vi "Total DAQ Link Data.vi"(9 "2 LBCB Archiving Mode":bool, 10 "Use Hold":bool, 11 "Number of LBCBs":T1) -> (1 "External Sensors":dbl[](array[numeric]), 2 "Act Data":dbl[](array[numeric]), 3 "Cart Data":dbl[](array[numeric]))   [LabVIEW 2009]
uses:
  Data Access Objects/Application/Number Of LBCBs.ctl
  Cartesian Measurment Actions.ctl
  Data Access Objects/Metadata/LBCB Number.ctl
  Data Access Objects/Metadata/DAO Actions.ctl
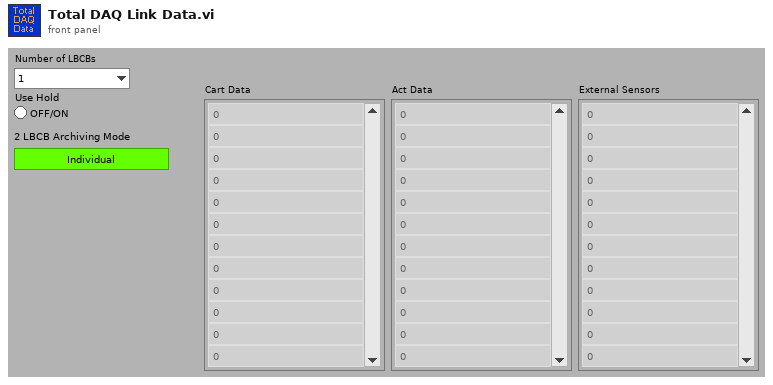
[diagram p1: front panel]
types:
  T1 = typedef "Number Of LBCBs.ctl" = enum16{"1", "2"}
  T2 = typedef "Cartesian Measurment Actions.ctl" = enum16{"Set Data", "Get", "Init", "Set Offsets"}
  T3 = typedef "LBCB Number.ctl" = enum16{"LBCB1", "LBCB2"}
  T4 = typedef "DAO Actions.ctl" = enum16{"Init", "Get", "Set"}
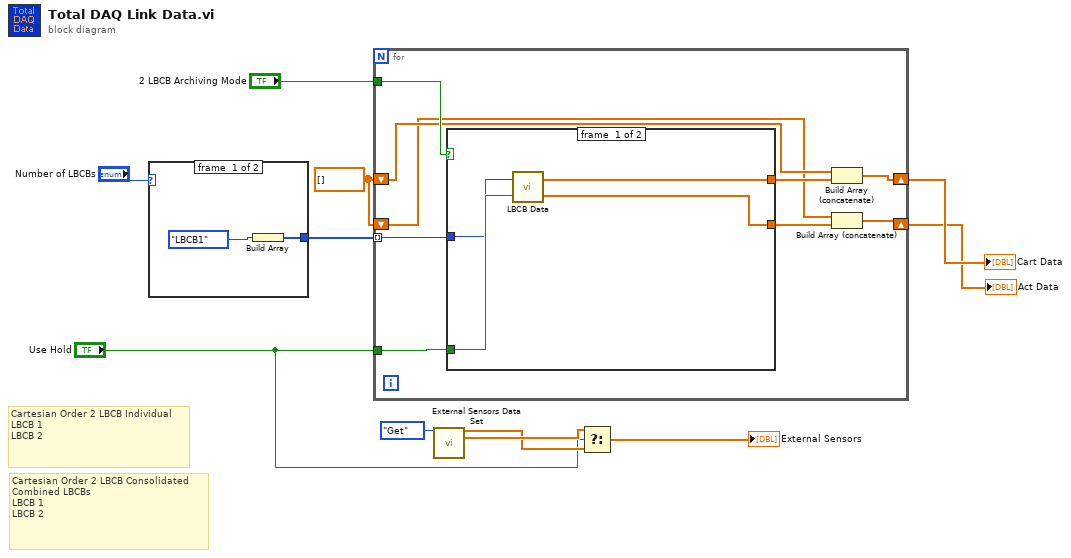
[diagram p0: block diagram]
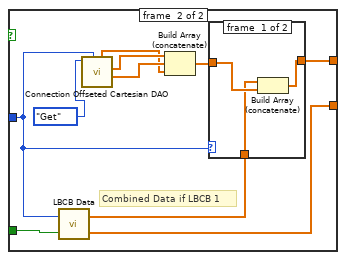
[diagram p2: hidden frame]
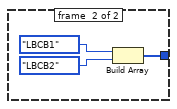
[diagram p4: hidden frame]
diagram:
  w8 = dbl[] [] ("Cart Data")
  # "Cartesian Order 2 LBCB Consolidated\nCombined LBCBs\nLBCB 1\nLBCB 2"
  # "Cartesian Order 2 LBCB Individual\nLBCB 1\nLBCB 2"
  n1 = case shown="\"1\", Default" "Number of LBCBs" {
    tunnel: [w12 w14] -> w10
    frame #0 {
      n2 = Build Array(LBCB_Number."LBCB1" ("LBCB Number")) -> (w12:T3[])
    }
    frame #1 {
      n3 = Build Array(LBCB_Number."LBCB1" ("LBCB Number"), LBCB_Number."LBCB2" ("LBCB Number")) -> (w14:T3[])
    }
  }
  n4 = for {
    tunnel: w10 -> [w23] mode=indexing
    tunnel: "Use Hold" -> [w25]
    tunnel: "2 LBCB Archiving Mode" -> [w21]
    shift-right: [w20] -> w7
    shift-left: w8 -> [w19]
    shift-right: [w18] -> w6
    shift-left: w8 -> [w17]
    n5 = case shown="True" w21 {
      tunnel: w25 -> [w29 w39]
      tunnel: [w28 w38] -> w24
      tunnel: w23 -> [w27 w33]
      tunnel: [w26 w30] -> w22
      frame #0 {
        n6 = call "LBCB Data.vi"("Use Hold"=w29, "LBCB Number"=w27) -> ("Act Data"=w28:dbl[], "Cart Data"=w26:dbl[])
      }
      frame #1 {
        # "Combined Data if LBCB 1"
        n7 = call "LBCB Data.vi"("Use Hold"=w39, "LBCB Number"=w33) -> ("Act Data"=w38:dbl[], "Cart Data"=w31:dbl[])
        n8 = call "Connection Offseted Cartesian DAO.vi"("LBCB Number"=w33, "DAO Actions"=DAO_Actions."Get") -> ("CO Disp Out"=w35:dbl[], "CO Cmd Out"=w36:dbl[], "CO Forces Out"=w34:dbl[])  [unwired: 6 in, 1 out]
        n9 = Build Array (concatenate)(w36, w35, w34) -> (w32:dbl[])
        n10 = case shown="\"LBCB1\"" w33 {
          tunnel: w32 -> [w42 w43]
          tunnel: w31 -> [w41 _]
          tunnel: [w40 w43] -> w30
          frame #0 {
            n11 = Build Array (concatenate)(w41, w42) -> (w40:dbl[])
          }
          frame #1 {
          }
        }
      }
    }
    n12 = Build Array (concatenate)(w19, w22) -> (w20:dbl[])
    n13 = Build Array (concatenate)(w17, w24) -> (w18:dbl[])
  }
  "Cart Data" <- w7
  "Act Data" <- w6
  n14 = call "External Sensors Data Set.vi"("Measurement Actions"=Cartesian_Measurment_Actions."Get") -> ("Data Out"=w3:dbl[], "Hold Data Out"=w4:dbl[])  [unwired: 10 in, 3 out]
  n15 = Select(t=w4, s="Use Hold", f=w3) -> (s? t:f=→"External Sensors":dbl[])
